vi "I2C L298P Motor Drive.vi"() -> ()   [LabVIEW 2020, in "CTI-Scratchpad.lvlib"]
uses:
  CTI-Scratchpad.lvlib
  CTI/Identity.ctl
  CTI/Error Reporting.ctl
  CTI/GPIO Number.ctl
  CTI/I2C Number.ctl
  CTI-Peripheral/Motor Controller/Base/Direction.ctl
  CTI/Session/Session.lvclass
  CTI-Peripheral/Motor Controller/Grove I2C L298P Motor Drive.lvclass
  CTI/VisaComms/VisaComms.lvclass
  CTI/CTI.lvlib
  CTI-Peripheral/Motor Controller/Base/Motor Controller.lvclass
panel:
  in  "Speed":i16(slide) scale=-100.0..100.0
  in  "Steering":i8(slide) scale=-100.0..100.0
  in  "M2":i16(slide) scale=-255.0..255.0
  in  "M1":i16(slide) scale=-255.0..255.0
  out "loop":i32
  in  "stop":bool
  out "Identity":T1
  in  "Grove Connector":enum16{"I2C0", "I2C1"}(ring)
  out "error out":errorcluster
  in  "Port":refnum<visa-resource-name>="COM6"
  # "https://wiki.seeedstudio.com/Grove-I2C-Motor-Driver-L298P/"
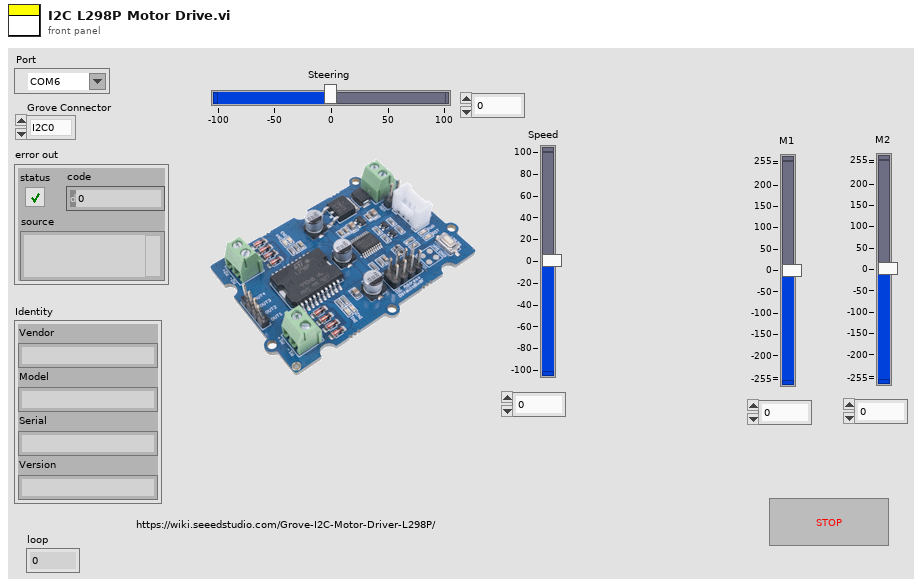
[diagram p1: front panel]
types:
  T1 = typedef "CTI.lvlib/Identity.ctl" = cluster{"Vendor":string, "Model":string, "Serial":string, "Version":string}
  T2 = typedef "CTI.lvlib/Error Reporting.ctl" = enum16{"Minimal", "Moderate", "Full"}
  T3 = typedef "CTI.lvlib/I2C Number.ctl" = i8
  T4 = typedef "CTI.lvlib/GPIO Number.ctl" = i8
  T5 = typedef "CTI-Peripheral.lvlib/Motor Controller.lvclass/Direction.ctl" = enum16{"No Direction - Error", "Clockwise (CW)", "Anti-Clockwise (ACW)"}
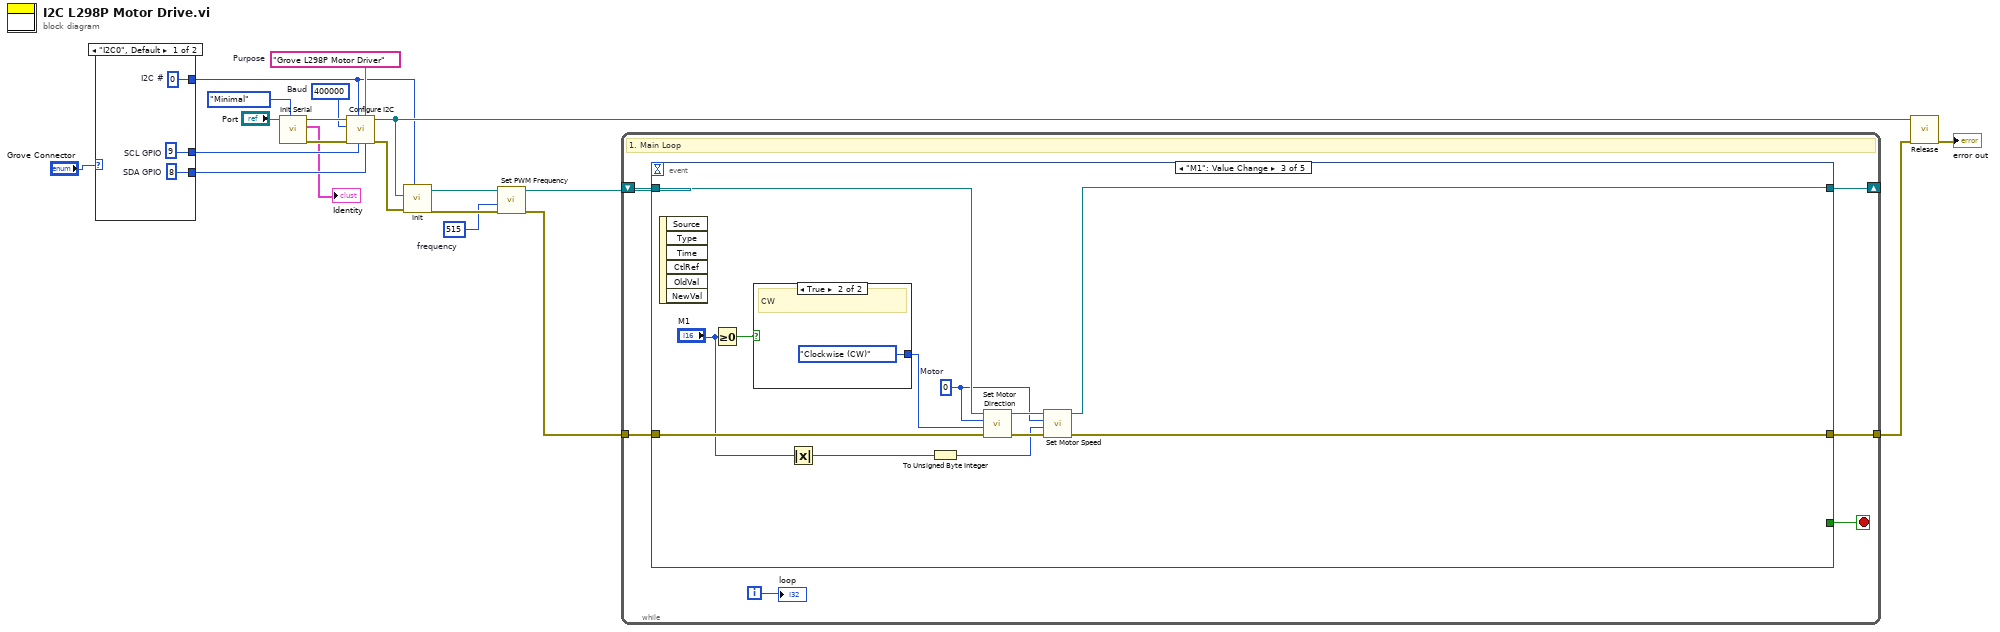
[diagram p0: block diagram]
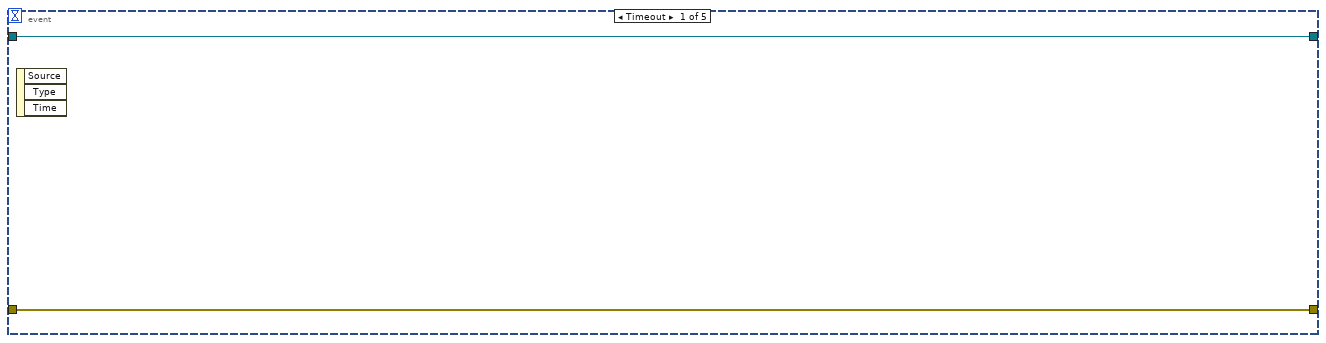
[diagram p2: hidden frame]
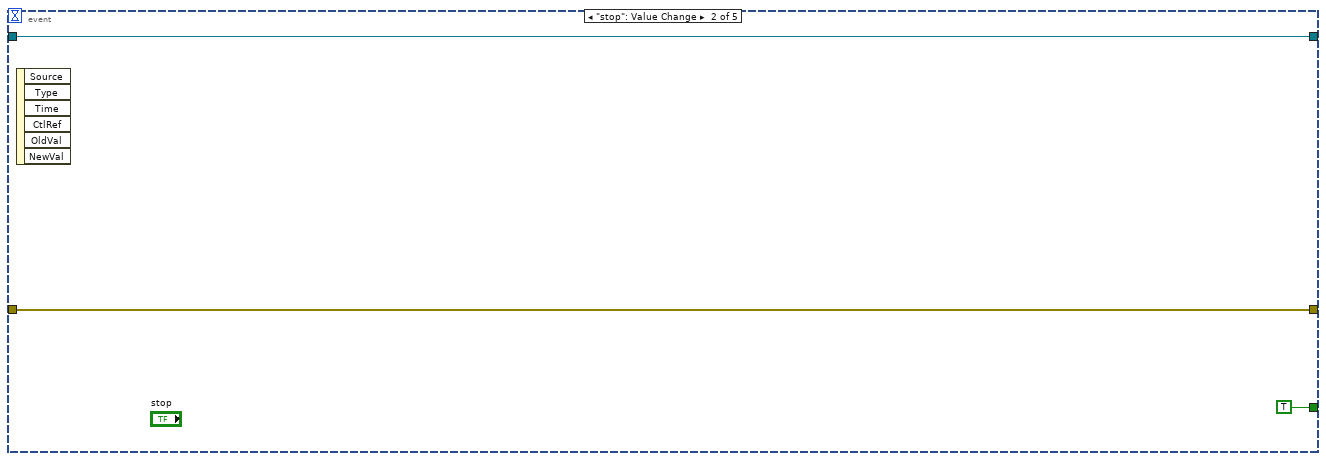
[diagram p3: hidden frame]
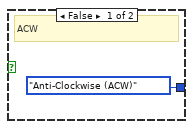
[diagram p4: hidden frame]
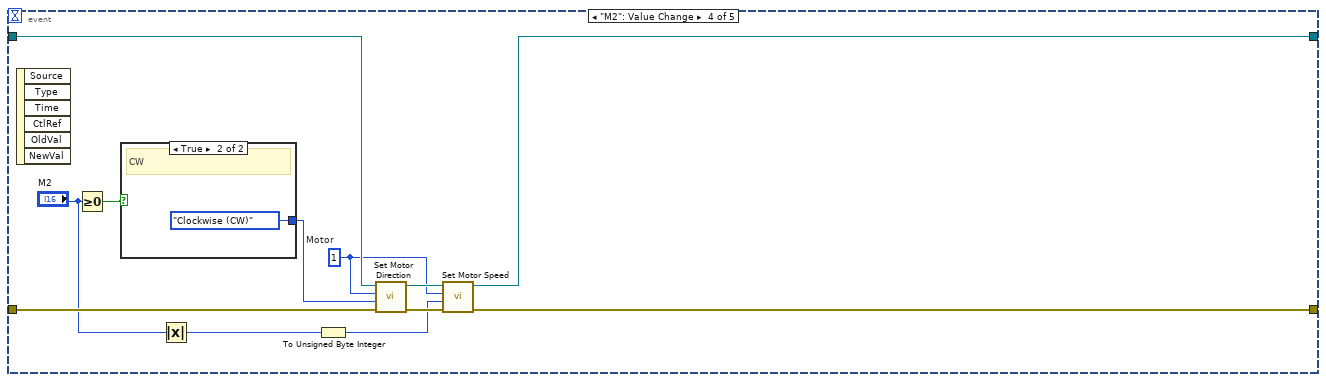
[diagram p5: hidden frame]
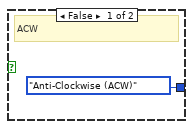
[diagram p6: hidden frame]
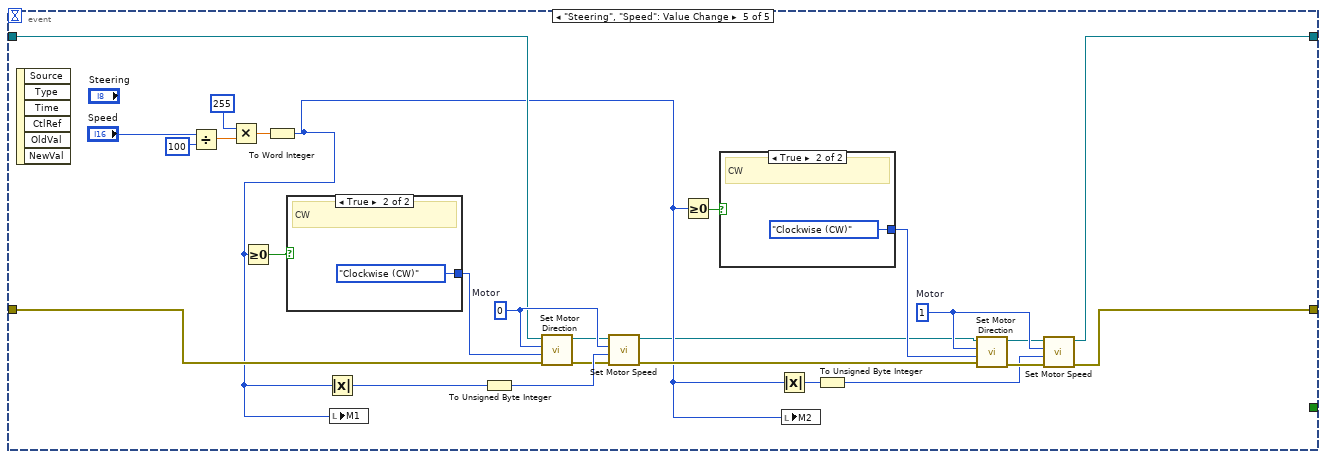
[diagram p7: hidden frame]
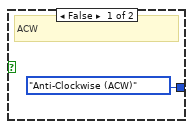
[diagram p8: hidden frame]
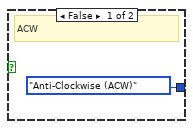
[diagram p9: hidden frame]
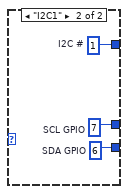
[diagram p10: hidden frame]
diagram:
  w1 = u16 515  # frequency
  w15 = "Grove L298P Motor Driver"  # Purpose
  w16 = u32 400000  # Baud
  n1 = case shown="\"I2C0\", Default" "Grove Connector" {
    tunnel: [w23 w26] -> w13
    tunnel: [w22 w25] -> w12
    tunnel: [w21 w24] -> w7
    frame "I2C0", Default {
      w21 = T3 0  # I2C #
      w22 = T4 8  # SDA GPIO
      w23 = T4 9  # SCL GPIO
    }
    frame "I2C1" {
      w24 = T3 1  # I2C #
      w25 = T4 6  # SDA GPIO
      w26 = T4 7  # SCL GPIO
    }
  }
  n2 = call "Init Serial.vi"("Error Checking (Full)"=Error_Reporting."Minimal", "VISA resource name in"="Port") -> ("error out"=w17:errorcluster, "Identity"=→"Identity":T1, "Session"=w18:refnum<class "Session.lvclass">)  [unwired: 7 in]
  n3 = call "Configure I2C.vi"("SDA GPIO"=w12, "Purpose (\"I2C\")"=w15, "SCL GPIO"=w13, "I2C #"=w7, "error in (no error)"=w17, "Baud"=w16, "Session in"=w18) -> ("error out"=w6:errorcluster, "Session out"=w8:refnum<class "Session.lvclass">)  [unwired: 3 in]
  n4 = call "Init.vi"("I2C #"=w7, "error in (no error)"=w6, "Session In"=w8) -> ("error out"=w4:errorcluster, "Grove I2C L298P Motor Drive Out"=w5:refnum<class "Grove I2C L298P Motor Drive.lvclass">)  [unwired: 7 in]
  n5 = call-dynamic "Set PWM Frequency.vi"("error in (no error)"=w4, "frequency"=w1, "Grove I2C L298P Motor Drive in"=w5) -> ("error out"=w2:errorcluster, "Grove I2C L298P Motor Drive out"=w3:refnum<class "Grove I2C L298P Motor Drive.lvclass">)  [unwired: 7 in]
  n6 = while {
    tunnel: w2 -> [w31]
    tunnel: [w29] -> w10
    shift-right: [w27] -> _
    shift-left: w3 -> [w32]
    i -> [w30]
    stop <- w28 stop-if-true
    # "1. Main Loop"
    n7 = event shown="[2] \"M1\": Value Change" {
      selector: _ -> [_ _ _ _ _]
      dyn-events: _ -> [_ _ _ _ _]
      timeout: _ -> [_ _ _ _ _]
      tunnel: w32 -> [w33 w35 w48 w62 w80]
      tunnel: w31 -> [w34 w36 w49 w63 w86]
      tunnel: [w34 w36 w39 w54 w77] -> w29
      tunnel: [_ TRUE _ _ _] -> w28
      tunnel: [w33 w35 w38 w52 w66] -> w27
      event Timeout {
        n8 = event-data() -> ()  [unwired: 1 in, 3 out]
      }
      event "stop": Value Change {
        n9 = event-data() -> ()  [unwired: 1 in, 6 out]
      }
      event "M1": Value Change {
        w43 = u16 0  # Motor
        n10 = event-data() -> ()  [unwired: 1 in, 6 out]
        n11 = Greater Or Equal To 0?(x="M1") -> (x >= 0?=w47:bool)
        n12 = case shown="True" w47 {
          tunnel: [Direction."Anti-Clockwise (ACW)" ("Direction") Direction."Clockwise (CW)" ("Direction")] -> w46
          frame False {
            # "ACW"
          }
          frame True {
            # "CW"
          }
        }
        n13 = Absolute Value(x="M1") -> (abs(x)=w40:i16)
        n14 = To Unsigned Byte Integer(number=w40) -> (unsigned 8bit integer=w41:u8)
        n15 = call-dynamic "Set Motor Direction.vi"("error in (no error)"=w49, "Direction"=w46, "Motor"=w43, "Grove I2C L298P Motor Drive in"=w48) -> ("error out"=w45:errorcluster, "Grove I2C L298P Motor Drive out"=w44:refnum<class "Grove I2C L298P Motor Drive.lvclass">)  [unwired: 6 in]
        n16 = call-dynamic "Set Motor Speed.vi"("error in (no error)"=w45, "Speed"=w41, "Motor"=w43, "Grove I2C L298P Motor Drive in"=w44) -> ("error out"=w39:errorcluster, "Grove I2C L298P Motor Drive out"=w38:refnum<class "Grove I2C L298P Motor Drive.lvclass">)  [unwired: 6 in]
      }
      event "M2": Value Change {
        w57 = u16 1  # Motor
        n17 = event-data() -> ()  [unwired: 1 in, 6 out]
        n18 = Greater Or Equal To 0?(x="M2") -> (x >= 0?=w61:bool)
        n19 = case shown="True" w61 {
          tunnel: [Direction."Anti-Clockwise (ACW)" ("Direction") Direction."Clockwise (CW)" ("Direction")] -> w60
          frame False {
            # "ACW"
          }
          frame True {
            # "CW"
          }
        }
        n20 = Absolute Value(x="M2") -> (abs(x)=w55:i16)
        n21 = To Unsigned Byte Integer(number=w55) -> (unsigned 8bit integer=w56:u8)
        n22 = call-dynamic "Set Motor Direction.vi"("error in (no error)"=w63, "Direction"=w60, "Motor"=w57, "Grove I2C L298P Motor Drive in"=w62) -> ("error out"=w59:errorcluster, "Grove I2C L298P Motor Drive out"=w58:refnum<class "Grove I2C L298P Motor Drive.lvclass">)  [unwired: 6 in]
        n23 = call-dynamic "Set Motor Speed.vi"("error in (no error)"=w59, "Speed"=w56, "Motor"=w57, "Grove I2C L298P Motor Drive in"=w58) -> ("error out"=w54:errorcluster, "Grove I2C L298P Motor Drive out"=w52:refnum<class "Grove I2C L298P Motor Drive.lvclass">)  [unwired: 6 in]
      }
      event "Steering", "Speed": Value Change {
        w85 = u16 1  # Motor
        w87 = u16 0  # Motor
        n24 = event-data() -> ()  [unwired: 1 in, 6 out]
        n25 = Divide(x="Speed", y=u8 100) -> (x/y=w75:dbl)
        n26 = Multiply(x=i16 255 ("Value (Signaling)"), y=w75) -> (x*y=w74:dbl)
        n27 = To Word Integer(number=w74) -> (16bit integer=w70:i16)
        n28 = Greater Or Equal To 0?(x=w70) -> (x >= 0?=w90:bool)
        n29 = case shown="True" w90 {
          tunnel: [Direction."Anti-Clockwise (ACW)" ("Direction") Direction."Clockwise (CW)" ("Direction")] -> w89
          frame False {
            # "ACW"
          }
          frame True {
            # "CW"
          }
        }
        n30 = Absolute Value(x=w70) -> (abs(x)=w88:i16)
        n31 = local write "M1"(w70) -> ()
        n32 = To Unsigned Byte Integer(number=w88) -> (unsigned 8bit integer=w72:u8)
        n33 = call-dynamic "Set Motor Direction.vi"("error in (no error)"=w86, "Direction"=w89, "Motor"=w87, "Grove I2C L298P Motor Drive in"=w80) -> ("error out"=w69:errorcluster, "Grove I2C L298P Motor Drive out"=w68:refnum<class "Grove I2C L298P Motor Drive.lvclass">)  [unwired: 6 in]
        n34 = call-dynamic "Set Motor Speed.vi"("error in (no error)"=w69, "Speed"=w72, "Motor"=w87, "Grove I2C L298P Motor Drive in"=w68) -> ("error out"=w82:errorcluster, "Grove I2C L298P Motor Drive out"=w67:refnum<class "Grove I2C L298P Motor Drive.lvclass">)  [unwired: 6 in]
        n35 = Greater Or Equal To 0?(x=w70) -> (x >= 0?=w81:bool)
        n36 = case shown="True" w81 {
          tunnel: [Direction."Anti-Clockwise (ACW)" ("Direction") Direction."Clockwise (CW)" ("Direction")] -> w79
          frame False {
            # "ACW"
          }
          frame True {
            # "CW"
          }
        }
        n37 = Absolute Value(x=w70) -> (abs(x)=w78:i16)
        n38 = local write "M2"(w70) -> ()
        n39 = To Unsigned Byte Integer(number=w78) -> (unsigned 8bit integer=w71:u8)
        n40 = call-dynamic "Set Motor Direction.vi"("error in (no error)"=w82, "Direction"=w79, "Motor"=w85, "Grove I2C L298P Motor Drive in"=w67) -> ("error out"=w83:errorcluster, "Grove I2C L298P Motor Drive out"=w84:refnum<class "Grove I2C L298P Motor Drive.lvclass">)  [unwired: 6 in]
        n41 = call-dynamic "Set Motor Speed.vi"("error in (no error)"=w83, "Speed"=w71, "Motor"=w85, "Grove I2C L298P Motor Drive in"=w84) -> ("error out"=w77:errorcluster, "Grove I2C L298P Motor Drive out"=w66:refnum<class "Grove I2C L298P Motor Drive.lvclass">)  [unwired: 6 in]
      }
    }
    "loop" <- w30
  }
  n42 = call-dynamic "Release.vi"("error in (no error)"=w10, "Session in"=w8) -> ("error out"=→"error out":errorcluster)  [unwired: 9 in]
